vi "FunctDataMgr.Read Result Data.vi"(8 "error in (no error)":errorcluster, 11 "FunctDataMgr in":refnum<class "FunctDataMgr.lvclass">) -> (0 "error out":errorcluster, 1 "Num":T5[](array[typedef]) {"Status" items=["LOG", "PASS", "FAIL", "ERROR"]}, 2 "Attr":T7[](array[typedef]) {"Status" items=["LOG", "PASS", "FAIL", "ERROR"]}, 3 "FunctDataMgr out":refnum<class "FunctDataMgr.lvclass">, 4 "Result Info":T3={"State"=enum."Passing", "Code"=0, "Description"=""}, 5 "Meas":T1[](array[typedef]) {"Status" items=["LOG", "PASS", "FAIL", "ERROR"]})   [LabVIEW 2024, in "FunctDataMgr.lvclass"]
uses:
  FunctDataMgr.lvclass
  Results/Result.Attribute.ctl
  Results/Result.Measurement and Attribute Item Status.ctl
  Results/Result.Numeric.ctl
  Results/Result.Limit Type.ctl
  <vilib>/KATE/SeqMgr/SeqMgr.Result Info.ctl
  <vilib>/KATE/SeqMgr/SeqMgr.Result State Enum.ctl
  Results/Result.Measurement Item.ctl
  FunctDataMgr.lvclass/FunctDataMgr.ctl
  <vilib>/KATE/SeqMgr/SeqMgr.lvlib
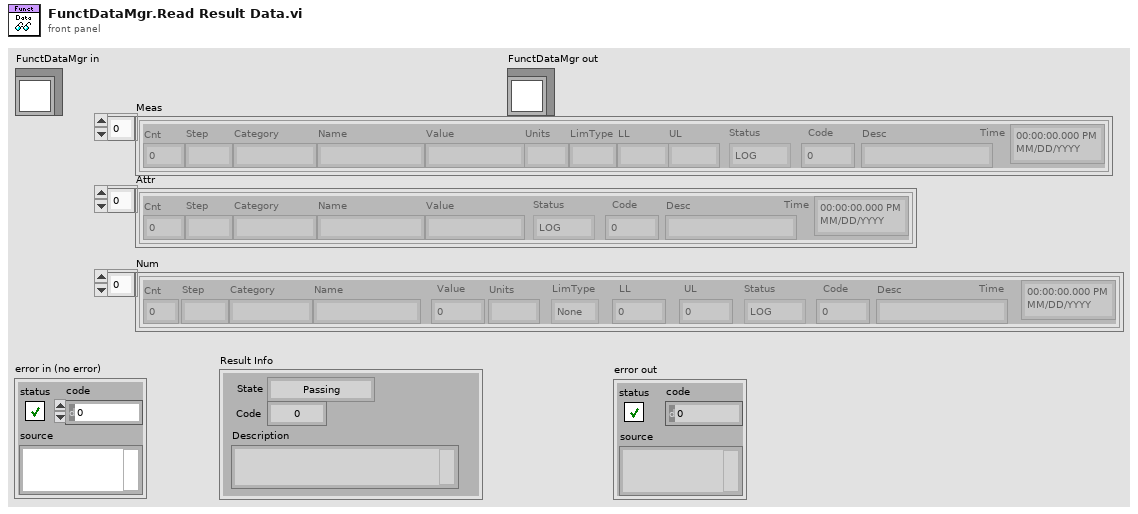
[diagram p1: front panel]
types:
  T1 = typedef "Result.Measurement Item.ctl" = cluster{"Cnt":i32, "Step":string, "Category":string, "Name":string, "Value":string, "Units":string, "LimType":string, "LL":string, "UL":string, "Status":T2, "Code":i32, "Desc":string, "Time":timestamp}
  T2 = typedef "Result.Measurement and Attribute Item Status.ctl" = i32
  T3 = typedef "KATE_Lib.lvlib/SeqMgr.lvlib/SeqMgr.Result Info.ctl" = cluster{"State":T4, "Code":i32, "Description":string}
  T4 = typedef "KATE_Lib.lvlib/SeqMgr.lvlib/SeqMgr.Result State Enum.ctl" = enum16{"None", "Passing", "Failing", "PASS", "FAIL", "ABORT", "ERROR"}
  T5 = typedef "Result.Numeric.ctl" = cluster{"Cnt":i32, "Step":string, "Category":string, "Name":string, "Value":dbl, "Units":string, "LimType":T6, "LL":dbl, "UL":dbl, "Status":T2, "Code":i32, "Desc":string, "Time":timestamp}
  T6 = typedef "Result.Limit Type.ctl" = enum16{"None", "EQ", "NE", "GT", "LT", "GE", "LE", "GTLT", "GELE", "GELT", "GTLE", "LTGT", "LEGE", "LEGT", "LTGE", "Contains", "NotContains"}
  T7 = typedef "Result.Attribute.ctl" = cluster{"Cnt":i32, "Step":string, "Category":string, "Name":string, "Value":string, "Status":T2, "Code":i32, "Desc":string, "Time":timestamp}
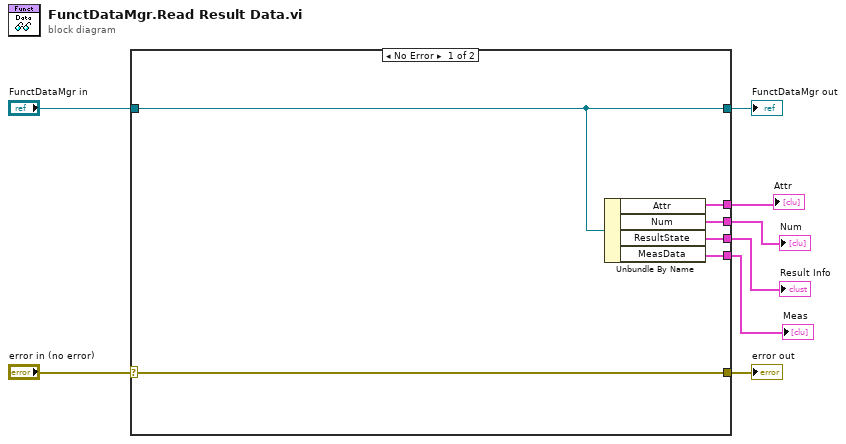
[diagram p0: block diagram]
diagram:
  n1 = case shown="No Error" "error in (no error)" {
    selector: "error in (no error)" -> [w14 w16]
    tunnel: [w14 w16] -> w7
    tunnel: [w13 w15] -> w5
    tunnel: "FunctDataMgr in" -> [w13 w15]
    tunnel: [w12 _] -> w4
    tunnel: [w11 _] -> w3
    tunnel: [w10 _] -> w2
    tunnel: [w9 _] -> w1
    frame No Error {
      n2 = Unbundle By Name(w13) -> ("Attr"=w12:T7[], "Num"=w11:T5[], "ResultState"=w10:T3, "MeasData"=w9:T1[])
    }
    frame Error {
    }
  }
  "error out" <- w7
  "FunctDataMgr out" <- w5
  "Attr" <- w4
  "Num" <- w3
  "Result Info" <- w2
  "Meas" <- w1
